vi "set wait.vi"(8 "error in (no error)":errorcluster, 10 "wait":u32[](array[numeric]), 11 "TestInterface in":refnum<class "TestInterface.lvclass">) -> (0 "error out":errorcluster, 3 "TestInterface out":refnum<class "TestInterface.lvclass">)   [LabVIEW 2013, in "TestInterface.lvclass"]
uses:
  TestInterface.lvclass
  TestInterface.lvclass/TestInterface.ctl
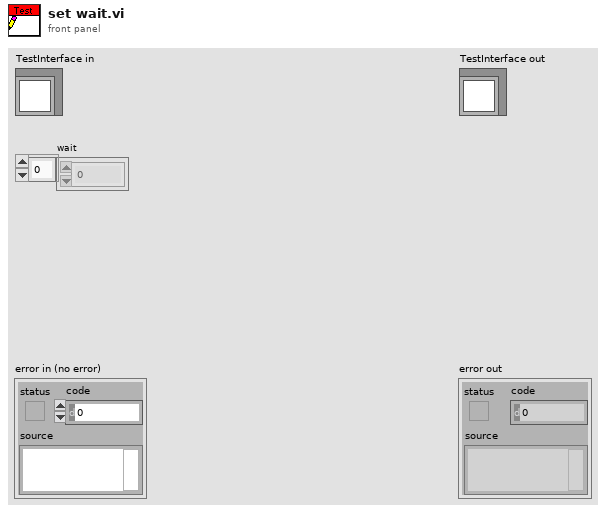
[diagram p1: front panel]
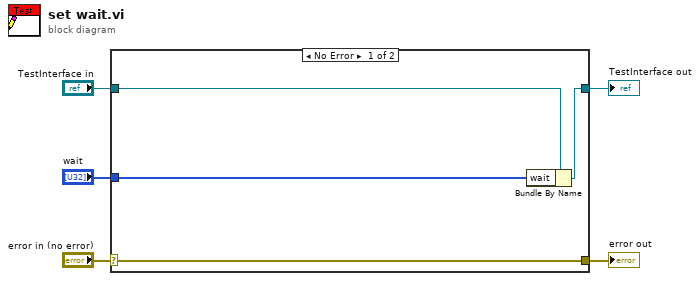
[diagram p0: block diagram]
diagram:
  n1 = case shown="No Error" "error in (no error)" {
    selector: "error in (no error)" -> [w9 w10]
    tunnel: [w9 w10] -> w4
    tunnel: [w7 w11] -> w2
    tunnel: "TestInterface in" -> [w8 w11]
    tunnel: "wait" -> [w6 _]
    frame No Error {
      n2 = Bundle By Name(cluster=w8, "wait"=w6) -> (w7:refnum<class "TestInterface.lvclass">)
    }
    frame Error {
    }
  }
  "error out" <- w4
  "TestInterface out" <- w2
